vi "Main5.vi"() -> ()   [LabVIEW 2014]
doc: "The myRIO Project template acquires acceleration data from the onboard accelerometer and displays the changes of acceleration values in a waveform chart."
uses:
  <vilib>/myRIO/Instrument Drivers/Onboard IO/AI/typedefs/AI Reference.ctl
  <vilib>/myRIO/Common/Instrument Driver Framework/Utilities/typedefs/myRIO Generic Hardware Reference.ctl
  <vilib>/myRIO/Common/Instrument Driver Framework/Utilities/typedefs/Hardware Version Enum.ctl
  <vilib>/myRIO/Common/Instrument Driver Framework/Utilities/typedefs/myRIO v1.0 Reference.ctl
  <vilib>/myRIO/Common/Instrument Driver Framework/Utilities/typedefs/Generic FPGA Reference.ctl
  <vilib>/myRIO/Common/Instrument Driver Framework/myRIO v1.0/AI/typedefs/AI Channels List.ctl
  <vilib>/myRIO/Common/Instrument Driver Framework/myRIO v1.0/AI/typedefs/AI Channels Enum.ctl
  <vilib>/myRIO/Common/Instrument Driver Framework/Utilities/typedefs/Analog Scaling Constants List.ctl
  <vilib>/myRIO/Common/Instrument Driver Framework/Utilities/typedefs/Analog Scaling Constants.ctl
  <vilib>/userdefined/High Color/nirio_resource_hc.ctl
  <vilib>/myRIO/Common/Instrument Driver Framework/Utilities/vis/Is FPGA Ref Available.vi
  <vilib>/myRIO/Common/Instrument Driver Framework/myRIO v1.0/AI/vis/myRIO v1.1 Open AI.vi
  <vilib>/myRIO/Instrument Drivers/Onboard IO/AI/vis/Read.vi
  <vilib>/myRIO/Common/Instrument Driver Framework/Utilities/vis/Validate Channels.vi
  <vilib>/myRIO/Common/Instrument Driver Framework/myRIO v1.0/AI/vis/myRIO v1.0 Reserve AI.vi
  <vilib>/myRIO/Common/Instrument Driver Framework/myRIO v1.0/AI/vis/myRIO v1.0 Build MUX Configuration AI.vi
  <vilib>/myRIO/Common/Instrument Driver Framework/myRIO v1.0/Resource Manager/vis/myRIO v1.0 Reserve Channel List.vi
  <vilib>/myRIO/Common/Instrument Driver Framework/myRIO v1.0/Resource Manager/vis/myRIO v1.0 Reserve Channel.vi
  <vilib>/myRIO/Common/Instrument Driver Framework/myRIO v1.0/Resource Manager/vis/myRIO v1.0 Unreserve Channel.vi
  <vilib>/myRIO/Common/Instrument Driver Framework/myRIO v1.0/Resource Manager/vis/myRIO v1.0 Build Mutex Name.vi
  <vilib>/Utility/VariantDataType/GetNumericInfo.vi
  <vilib>/Utility/error.llb/Error Cluster From Error Code.vi
  <vilib>/myRIO/Common/Instrument Driver Framework/myRIO v1.0/myRIO v1.1 Open.vi
  <vilib>/myRIO/Common/Instrument Driver Framework/myRIO v1.0/AI/vis/myRIO v1.0 Get Scaling Constants AI.vi
  <vilib>/myRIO/Common/Instrument Driver Framework/Utilities/vis/IO Manager.vi
  <vilib>/myRIO/Common/Instrument Driver Framework/Utilities/vis/Configuration Manager.vi
  <vilib>/myRIO/Common/Instrument Driver Framework/myRIO v1.0/myRIO v1.0 Close.vi
  <vilib>/myRIO/Common/Instrument Driver Framework/myRIO v1.0/AI/vis/myRIO v1.0 Read AI.vi
  <vilib>/myRIO/Express VI/Onboard IO/AI/AI Express VI.xnode
  <vilib>/myRIO/Instrument Drivers/Onboard IO/AI/vis/myRIO AI Open.xnode
  <vilib>/vision/driver/NI_Vision_Acquisition_Software.lvlib
  <vilib>/vision/NI_Vision_Development_Module.lvlib
  <vilib>/myRIO/Instrument Drivers/Onboard IO/AI/AI.lvlib
panel:
  out "Acceleration 4":dbl(graph)
  out "x*y":dbl
  out "Acceleration 3":dbl(graph)
  out "x-y":dbl=7.5880973321606575
  in  "y":dbl=15.0
  out "범위내?":bool=TRUE
  out "웨이브폼 차트 2":dbl(graph)=-0.0
  in  "3":u8=3
  in  "Controller 2":u8=2
  in  "Number of Erosion":i32=4
  in  "Red or Hue":cluster{i32, i32}(slide)={237, 15} scale=0.0..255.0
  in  "Threshold Color Mode":enum32{"RGB", "HSL"}(radio)=enum."HSL"
  in  "Green or Saturation":cluster{i32, i32}(slide)={104, 255} scale=0.0..255.0
  in  "Blue or Luminance":cluster{i32, i32}(slide)={0, 255} scale=0.0..255.0
  out "Image 2":T1(plugin-control)
  in  "Stop 2":bool
  out "Image":T1(plugin-control)
  in  "Camera Name":refnum<k21>="cam3" caption="IMAQdx Session"
  # "Control Motor"
  # "Read Encoder"
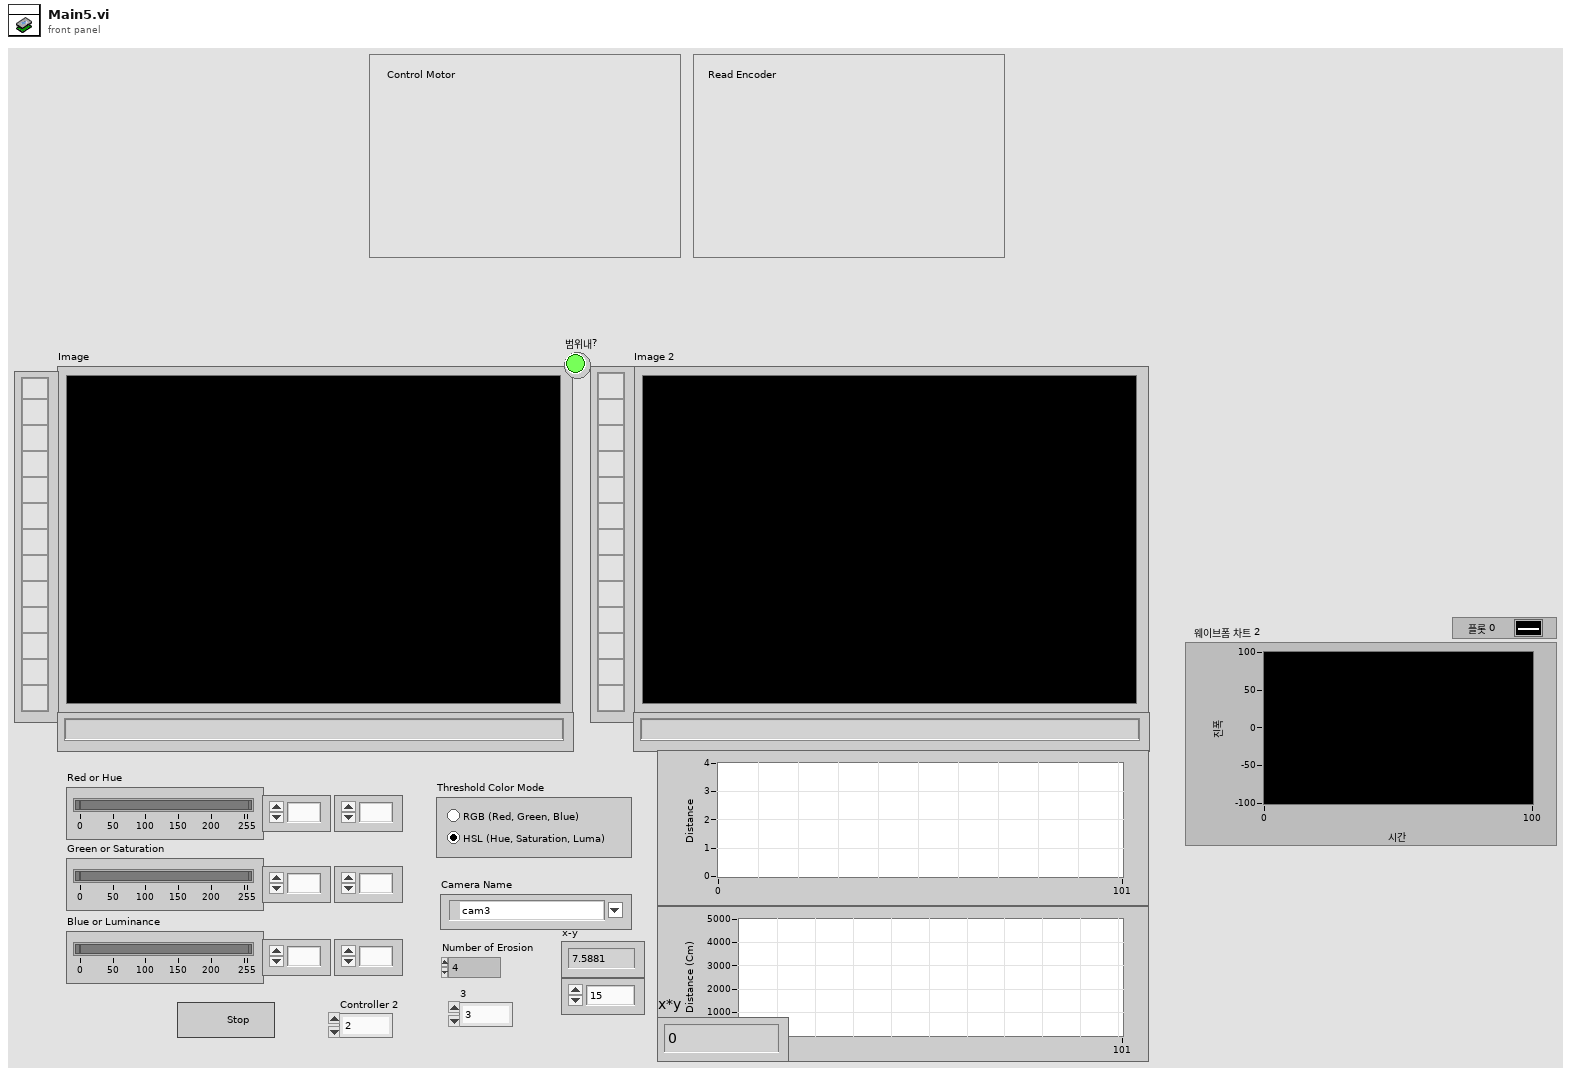
[diagram p1: front panel]
types:
  T1 = typedef "IMAQ Image.ctl" = refnum<image>
  T2 = typedef "AI.lvlib/AI Reference.ctl" = cluster{"myRIO Reference":T3, "AI Channels List":T7, "AI Scaling Constants List":T9}
  T3 = typedef "myRIO Generic Hardware Reference.ctl" = cluster{"myRIO Model":T4, "myRIO Hardware Reference":T5}
  T4 = typedef "Hardware Version Enum.ctl" = enum16{"Unknown", "myRIO-1900", "myRIO-1950"}
  T5 = typedef "myRIO v1.0 Reference.ctl" = cluster{"Generic FPGA Reference":T6, "Allow multiple opens":bool}
  T6 = typedef "Generic FPGA Reference.ctl" = refnum<k20>
  T7 = typedef "AI Channels List.ctl" = T8[]
  T8 = typedef "AI Channels Enum.ctl" = enum16{"Not Connected", "AudioIn/Left", "AudioIn/Right", "C/AI0", "C/AI1", "A/AI0", "A/AI1", "A/AI2", "A/AI3", "B/AI0", "B/AI1", "B/AI2", "B/AI3"}
  T9 = typedef "Analog Scaling Constants List.ctl" = T10[]
  T10 = typedef "Analog Scaling Constants.ctl" = cluster{"LSB Weight (Volts)":dbl, "Offset (Volts)":dbl, "Signed?":bool}
  T11 = typedef "nirio_resource_hc.ctl" = tag
  T12 = typedef "IMAQ Rectangle" = cluster{"Left":i32, "Top":i32, "Right":i32, "Bottom":i32, "Rotation":dbl}
  T13 = typedef "Image Type" = u32
  T14 = typedef "IMAQdx.ctl" = refnum<k21>
  T15 = cluster{"Global Rectangle":i32[], "Contours":cluster{"Contour Type":u32, "ROI Type":u32, "Points":i32[]}[]}
  T16 = cluster{"Area":dbl, "Number of Holes":dbl, "Bounding Rect":cluster{"Left":dbl, "Top":dbl, "Right":dbl, "Bottom":dbl}, "Center of Mass":cluster{"X":dbl, "Y":dbl}, "Orientation":dbl, "Dimensions":cluster{"Width":dbl, "Height":dbl}}[]
  T17 = cluster{"Area":dbl, "Number of Holes":dbl, "Bounding Rect":cluster{"Left":dbl, "Top":dbl, "Right":dbl, "Bottom":dbl}, "Center of Mass":cluster{"X":dbl, "Y":dbl}, "Orientation":dbl, "Dimensions":cluster{"Width":dbl, "Height":dbl}}
  T18 = cluster{"Left":dbl, "Top":dbl, "Right":dbl, "Bottom":dbl}
  T19 = typedef "ROI Descriptor" = cluster{"Global Rectangle":i32[], "Contours":cluster{"ID":enum32{"External", "Internal"}, "Type":u32, "Coordinates":i32[]}[]}
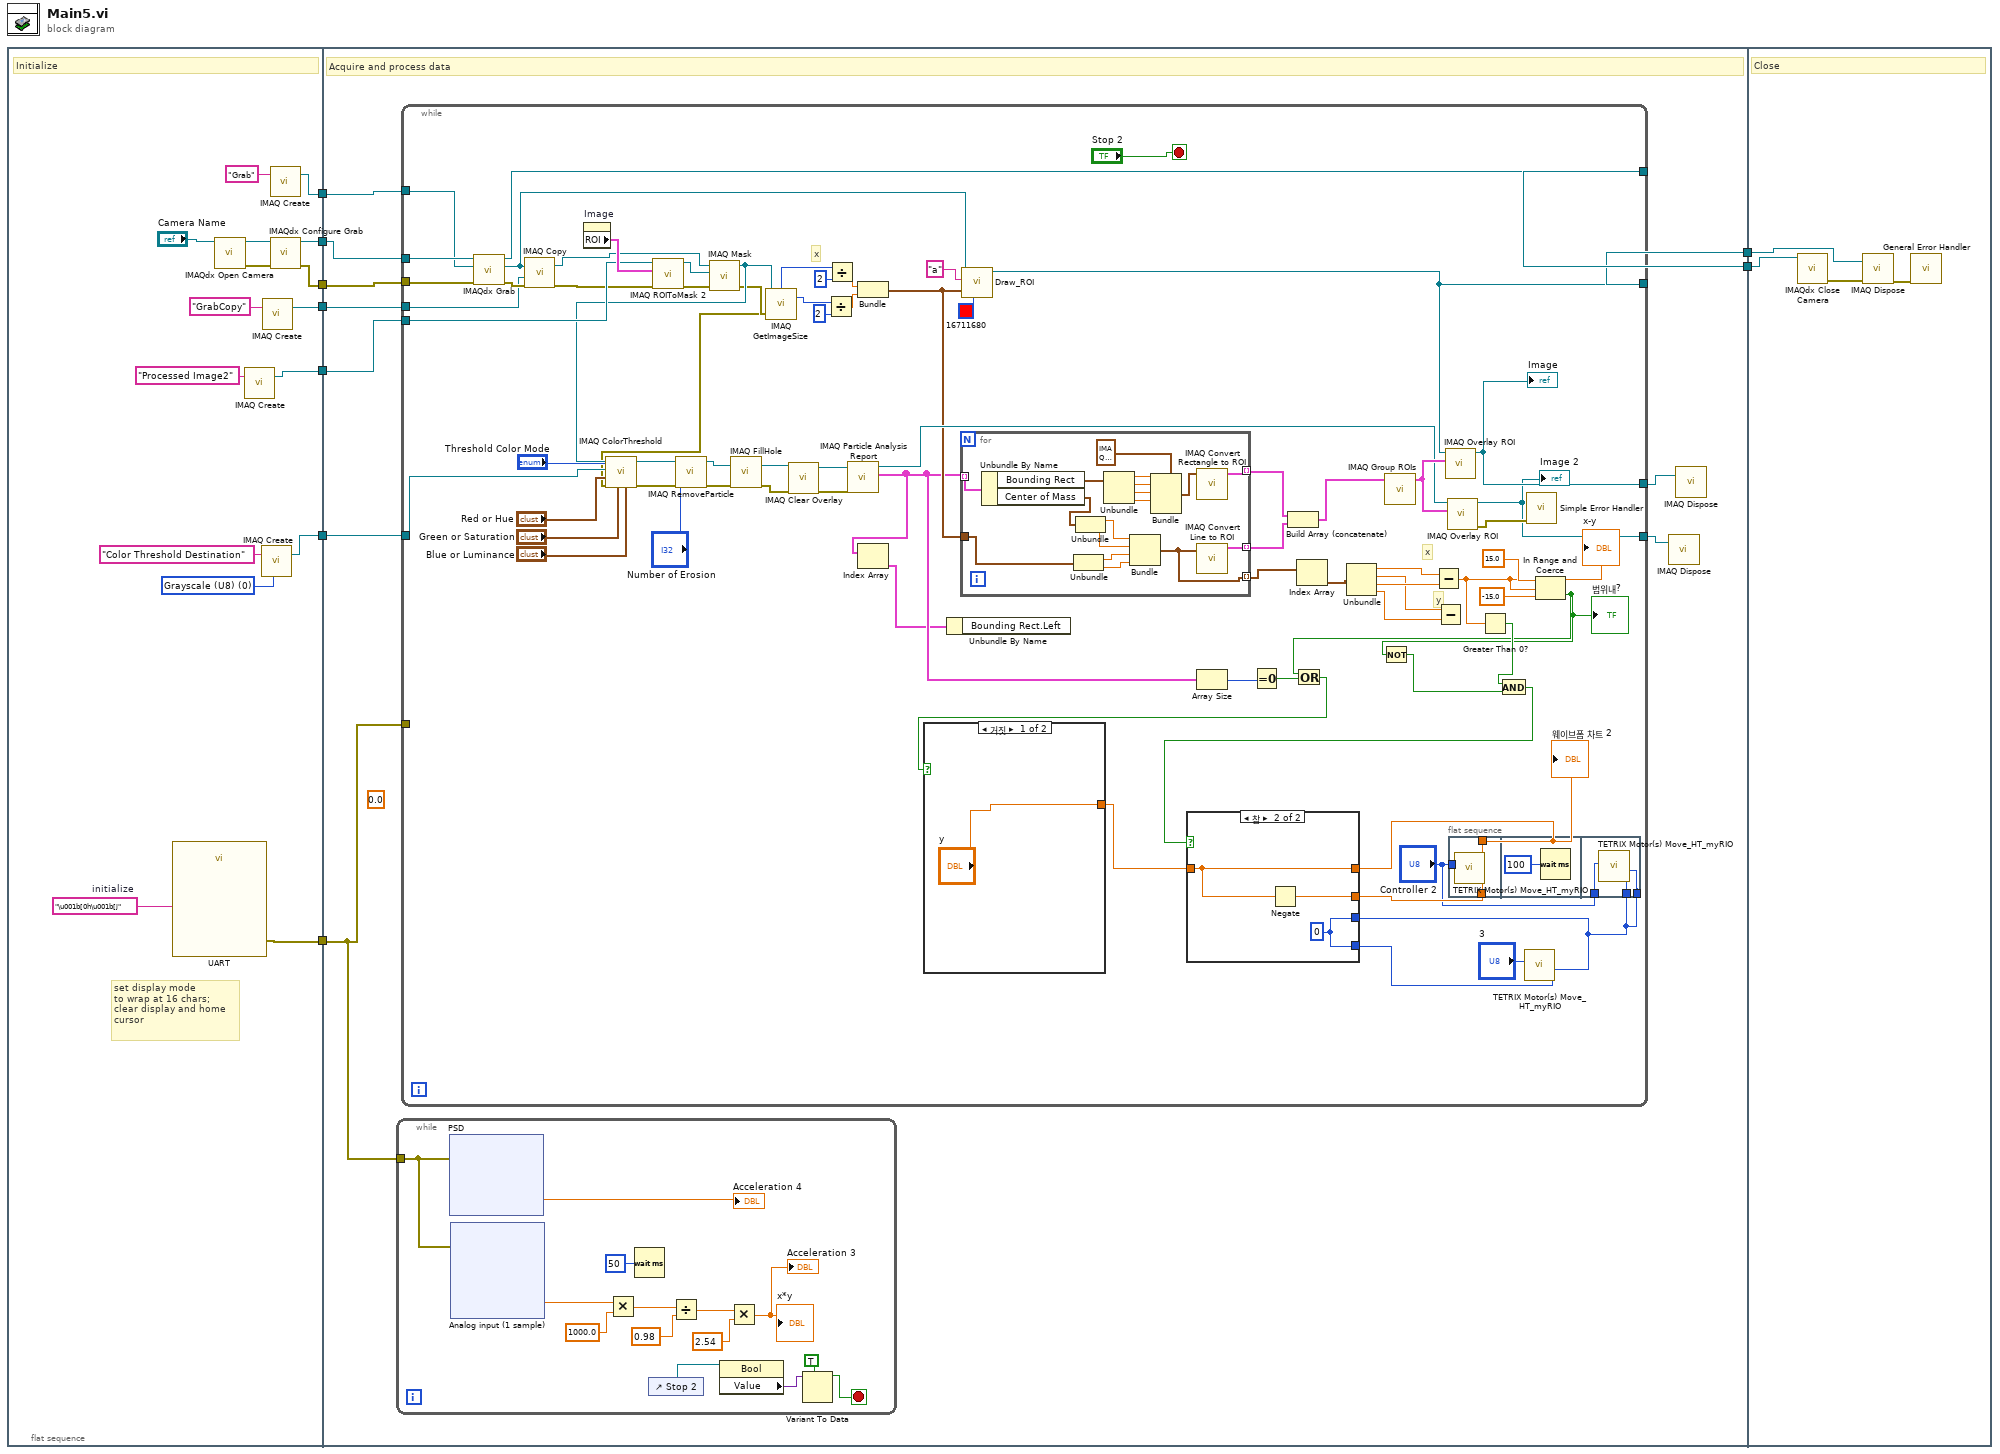
[diagram p0: block diagram]
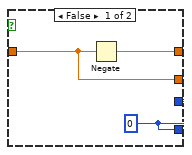
[diagram p2: hidden frame]
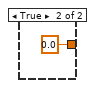
[diagram p3: hidden frame]
diagram:
  n1 = flat-sequence {
    tunnel: [w21] -> w9
    tunnel: [w20] -> w8
    tunnel: [w19] -> w7
    tunnel: [w17] -> w4
    tunnel: [w15] -> w3
    tunnel: [w14] -> w2
    tunnel: [w10] -> w1
    tunnel: w9 -> [w36]
    tunnel: w8 -> [w35]
    tunnel: w7 -> [w34]
    tunnel: [w28] -> w6
    tunnel: [w33] -> w5
    tunnel: w4 -> [w30]
    tunnel: w3 -> [w29]
    tunnel: w2 -> [w26]
    tunnel: w1 -> [w27]
    tunnel: w6 -> [w232]
    tunnel: w5 -> [w231]
    frame #0 {
      w12 = T13 0 items=["Grayscale (U8)", "Grayscale (I16)", "Grayscale (SGL)", "Complex (CSG)", "RGB (U32)", "HSL (U32)", "RGB (U64)", "Grayscale (U16)"] ("Image Type")
      w13 = "\u001b[0h\u001b[j"  # initialize
      # "set display mode\nto wrap at 16 chars;\nclear display and home\ncursor"
      # "Initialize"
      n2 = call "UART"("Characters to Write"=w13) -> ("error out"=w14:errorcluster)  [unwired: 25 in, 1 out]
      n3 = call <vilib>:"IMAQdx Open Camera.vi"("Session In"="Camera Name") -> ("error out"=w25:errorcluster, "Session Out"=w24:T14)  [unwired: 2 in, 7 out]
      n4 = call "IMAQ Create"("Image Name"="Processed Image2") -> ("New Image"=w17:T1)  [unwired: 3 in, 2 out]
      n5 = call "IMAQ Create"("Image Name"="Color Threshold Destination", "Image Type"=w12) -> ("New Image"=w10:T1)  [unwired: 3 in, 1 out]
      n6 = call "IMAQ Create"("Image Name"="GrabCopy") -> ("New Image"=w15:T1)  [unwired: 3 in, 2 out]
      n7 = call "IMAQ Create"("Image Name"="Grab") -> ("New Image"=w21:T1)  [unwired: 3 in, 2 out]
      n8 = call <vilib>:"IMAQdx Configure Grab.vi"("error in"=w25, "Session In"=w24) -> ("error out"=w19:errorcluster, "Session Out"=w20:T14)  [unwired: 8 out]
    }
    frame #1 {
      (unwired) 0.0 ("y")
      # "Acquire and process data"
      n9 = while {
        tunnel: w26 -> [w39]
        stop <- w47 stop-if-true
        n10 = xnode "PSD"("error in (no error)"=w39) -> ("C/AI0 (C/AI0 (AI0))"=→"Acceleration 4":dbl)  [unwired: 1 out]
        n11 = xnode "Analog input (1 sample)"("error in (no error)"=w39) -> ("UltraSonic (A/AI0 (Pin 3))"=w41:dbl)  [unwired: 1 out]
        n12 = Multiply(x=w41, y=1000.0) -> (x*y=w44:dbl)
        n13 = Wait (ms)(milliseconds to wait=u32 50 ("대기 시간(ms)")) -> ()  [unwired: 1 out]
        n14 = control-ref of="Stop 2"() -> (w50:refnum<vi>)
        n15 = Divide(x=w44, y=0.98) -> (x/y=w42:dbl)
        n16 = property class="Bool"(reference=w50) -> ("Value"=w49:variant)  [unwired: 1 in, 2 out]
        n17 = Multiply(x=w42, y=2.54) -> (x*y=→"x*y" →"Acceleration 3":dbl)
        n18 = Variant To Data(type=TRUE, Variant=w49) -> (data=w47:bool)  [unwired: 1 in, 1 out]
      }
      n19 = while {
        tunnel: [w195] -> w33
        tunnel: w34 -> [w197]
        tunnel: w35 -> [w198]
        tunnel: w36 -> [w196]
        tunnel: [w165] -> w32
        tunnel: [w164] -> w31
        tunnel: w30 -> [w187]
        tunnel: w29 -> [w173]
        tunnel: [w166] -> w28
        tunnel: w26 -> [_]
        tunnel: w27 -> [w155]
        stop <- "Stop 2" stop-if-true
        # "y"
        # "x"
        # "x"
        n20 = call <vilib>:"IMAQdx Grab.vi"("error in"=w197, "Image In"=w196, "Session In"=w198) -> ("error out"=w175:errorcluster, "Image Out"=w171:T1, "Session Out"=w195:T14)  [unwired: 1 in, 5 out]
        n21 = call "IMAQ Copy"("error in (no error)"=w175, "Image Dst"=w173, "Image Src"=w171) -> ("error out"=w174:errorcluster, "Image Dst Out"=w172:T1)  [unwired: 3 in]
        n22 = property on="Image" class="ImageControl"() -> ("ROI"=w189:T15)  [unwired: 2 in, 2 out]
        n23 = call "IMAQ ROIToMask 2"("error in (no error)"=w174, "ROI Descriptor"=w189, "Image"=w187) -> ("error out"=w185:errorcluster, "Image Out"=w186:T1)  [unwired: 6 in, 1 out]
        n24 = call "IMAQ Mask"("error in (no error)"=w185, "Image Mask"=w186, "Image Src"=w172) -> ("error out"=w163:errorcluster, "Image Dst Out"=w170:T1)  [unwired: 2 in]
        n25 = call "IMAQ GetImageSize"("Image"=w170, "error in (no error)"=w163) -> ("Y Resolution"=w180:i32, "X Resolution"=w183:i32, "error out"=w147:errorcluster)  [unwired: 2 in]
        n26 = call "IMAQ ColorThreshold"("Blue or Luma or Val or Inten Range"="Blue or Luminance", "Green or Sat Range"="Green or Saturation", "Color Mode"="Threshold Color Mode", "error in (no error)"=w147, "Red or Hue Range"="Red or Hue", "Image Dst"=w155, "Image Src"=w170) -> ("error out"=w148:errorcluster, "Image Dst Out"=w150:T1)  [unwired: 3 in]
        n27 = call "IMAQ RemoveParticle"("error in (no error)"=w148, "Number of Erosion"="Number of Erosion", "Image Src"=w150) -> ("error out"=w143:errorcluster, "Image Dst Out"=w144:T1)  [unwired: 7 in]
        n28 = call "IMAQ FillHole"("error in (no error)"=w143, "Image Src"=w144) -> ("error out"=w146:errorcluster, "Image Dst Out"=w145:T1)  [unwired: 4 in]
        n29 = call "IMAQ Clear Overlay"("error in (no error)"=w146, "Image"=w145) -> ("error out"=w184:errorcluster, "Image Out"=w191:T1)  [unwired: 1 in, 7 out]
        n30 = Divide(x=w180, y=2) -> (x/y=w178:dbl)
        n31 = Divide(x=w183, y=2) -> (x/y=w179:dbl)
        n32 = call "IMAQ Particle Analysis Report"("error in (no error)"=w184, "Image"=w191) -> ("Particle Reports (Pixels)"=w126:T16, "Image Out (duplicate)"=w190:T1)  [unwired: 4 in, 4 out]
        n33 = Bundle(w179, w178) -> (w169:cluster{dbl, dbl})  [unwired: 1 in]
        n34 = Index Array(array=w126) -> (element=w125:T17)  [unwired: 1 in]
        n35 = Unbundle By Name(w125) -> ()  [unwired: 1 out]
        n36 = for {
          tunnel: w126 -> [w230] mode=indexing
          tunnel: [w222] -> w168 mode=indexing
          tunnel: w169 -> [w218]
          tunnel: [w215] -> w162 mode=indexing
          tunnel: [w214] -> w161 mode=indexing
          n37 = Unbundle By Name(w230) -> ("Bounding Rect"=w228:T18, "Center of Mass"=w221:cluster{"X":dbl, "Y":dbl})
          n38 = Unbundle(w218) -> (w217:dbl, w216:dbl)
          n39 = Unbundle(w221) -> ("X"=w220:dbl, "Y"=w219:dbl)
          n40 = Unbundle(w228) -> ("Left"=w227:dbl, "Top"=w226:dbl, "Right"=w225:dbl, "Bottom"=w224:dbl)
          n41 = Bundle("X"=w220, "Y"=w219, w217, w216) -> (w214:cluster{"X":dbl, "Y":dbl, dbl, dbl})  [unwired: 1 in]
          n42 = Bundle(cluster=T12 {"Left"=0, "Top"=0, "Right"=0, "Bottom"=0, "Rotation"=0.0} ("Rectangle"), "Left"=w227, "Top"=w226, "Right"=w225, "Bottom"=w224) -> (w223:T12)  [unwired: 1 in]
          n43 = call "IMAQ Convert Rectangle to ROI"("Rectangle"=w223) -> ("ROI Descriptor"=w222:T19)  [unwired: 8 in, 1 out]
          n44 = call "IMAQ Convert Line to ROI"("Line"=w214) -> ("ROI Descriptor"=w215:T19)  [unwired: 8 in, 1 out]
        }
        n45 = call "Draw_ROI.vi"("Color"=u32 16711680, "클러스터"=w169, "Group"="a", "참조 번호 입력"=w171) -> ("참조 번호 출력"=w166:T1)  [unwired: 7 in]
        n46 = Array Size(array=w126) -> (size(s)=w192:i32)
        n47 = Equal To 0?(x=w192) -> (x = 0?=w132:bool)
        n48 = Build Array (concatenate)(w168, w162) -> (w167:T19[])
        n49 = Index Array(array=w161) -> (element=w160:cluster{"X":dbl, "Y":dbl, dbl, dbl})  [unwired: 1 in]
        n50 = Unbundle(w160) -> ("X"=w159:dbl, "Y"=w157:dbl, w158:dbl, w156:dbl)
        n51 = call "IMAQ Group ROIs"("ROI Descriptors"=w167) -> ("ROI Descriptor out"=w193:T19)  [unwired: 1 in, 3 out]
        n52 = Subtract(x=w159, y=w158) -> (x-y=w131:dbl)
        "x-y" <- w131
        n53 = Subtract(x=w157, y=w156) -> ()  [unwired: 1 out]
        n54 = call "IMAQ Overlay ROI"("ROI Descriptor"=w193, "Image"=w166) -> ("Image Out"=w165:T1)  [unwired: 4 in, 5 out]
        "Image" <- w165
        n55 = call "IMAQ Overlay ROI"("ROI Descriptor"=w193, "Image"=w190) -> ("error out"=w194:errorcluster, "Image Out"=w164:T1)  [unwired: 4 in, 4 out]
        "Image 2" <- w164
        n56 = flat-sequence {
          tunnel: "Controller 2" -> [w201]
          tunnel: w135 -> [w200]
          tunnel: w134 -> [w199]
          tunnel: "Controller 2" -> [w205]
          tunnel: w127 -> [w204]
          tunnel: w127 -> [w203]
          frame #0 {
            n57 = call <vilib>:"TETRIX Motor(s) Move_HT_myRIO.vi"("Motor 2 Power (-100 to 100)\n0 = Stop/Brake\n-128 = Stop/Coast"=w199, "Motor 1 Power (-100 to 100)\n0 = Stop/Brake\n-128 = Stop/Coast"=w200, "Controller Daisy Chain Position: 1 - 4"=w201) -> ()  [unwired: 6 in, 1 out]
          }
          frame #1 {
            n58 = Wait (ms)(milliseconds to wait=u32 100 ("대기 시간(ms)")) -> ()  [unwired: 1 out]
          }
          frame #2 {
            n59 = call <vilib>:"TETRIX Motor(s) Move_HT_myRIO.vi"("Motor 2 Power (-100 to 100)\n0 = Stop/Brake\n-128 = Stop/Coast"=w204, "Motor 1 Power (-100 to 100)\n0 = Stop/Brake\n-128 = Stop/Coast"=w203, "Controller Daisy Chain Position: 1 - 4"=w205) -> ()  [unwired: 6 in, 1 out]
          }
        }
        n60 = Greater Than 0?(x=w131) -> (x > 0?=w139:bool)
        n61 = call <vilib>:"Simple Error Handler.vi"("error in (no error)"=w194) -> ()  [unwired: 1 in, 8 out]
        n62 = In Range and Coerce(upper limit=15.0 ("상위 리미트"), x=w131, lower limit=-15.0 ("하위 리미트")) -> (In Range?=w129:bool)  [unwired: 1 out]
        "범위내?" <- w129
        n63 = Or(x=w129, y=w132) -> (x .or. y?=w138:bool)
        n64 = case shown="거짓" w138 {
          tunnel: ["y" 0.0 ("y")] -> w136
          frame False {
          }
          frame True {
          }
        }
        n65 = Not(x=w129) -> (.not. x?=w130:bool)
        n66 = And(x=w139, y=w130) -> (x .and. y?=w137:bool)
        n67 = case shown="참" w137 {
          tunnel: [w208 w211] -> w135
          tunnel: w136 -> [w207 w211]
          tunnel: [w207 w210] -> w134
          tunnel: [w206 w209] -> w133
          tunnel: [w206 w209] -> w127
          frame False {
            w206 = 0
            n68 = Negate(x=w207) -> (-x=w208:dbl)
          }
          frame True {
            w209 = 0
            n69 = Negate(x=w211) -> (-x=w210:dbl)
          }
        }
        "웨이브폼 차트 2" <- w135
        n70 = call <vilib>:"TETRIX Motor(s) Move_HT_myRIO.vi"("Motor 2 Power (-100 to 100)\n0 = Stop/Brake\n-128 = Stop/Coast"=w133, "Motor 1 Power (-100 to 100)\n0 = Stop/Brake\n-128 = Stop/Coast"=w127, "Controller Daisy Chain Position: 1 - 4"="3") -> ()  [unwired: 6 in, 1 out]
      }
      n71 = call "IMAQ Dispose"("Image"=w31) -> ()  [unwired: 5 in, 1 out]
      n72 = call "IMAQ Dispose"("Image"=w32) -> ()  [unwired: 5 in, 1 out]
    }
    frame #2 {
      # "Close"
      n73 = call <vilib>:"IMAQdx Close Camera.vi"("Session In"=w231) -> ("error out"=w234:errorcluster)  [unwired: 1 in, 9 out]
      n74 = call "IMAQ Dispose"("Image"=w232, "error in (no error)"=w234) -> ("error out"=w233:errorcluster)  [unwired: 4 in]
      n75 = call <vilib>:"General Error Handler.vi"("error in (no error)"=w233) -> ()  [unwired: 2 in, 13 out]
    }
  }
